vi "Curtin1_Plot.vi"(5 "Canvas 2":refnum<vi>, 6 "Force YRescale":bool, 7 "Settings":T2 {"mag/phase" items=["FRF", "rad phase unwrapped", "deg phase unwrapped", "rad phase wrapped", "deg phase wrapped", "White Plots", "MJ Map", "Real and Imaginary"]; "Bands" items=["No Bands", "", "Test2", "test3", "Test"]; "Smoothing" items=["No smoothing"=0, "1/4 semitone"=25, "1/2 semitone"=50, "1 semitone"=100, "2 semitones"=200, "Woodhouse"=19]; "View Type" items=["As measured", "Normalize", "Separate", "Complex Average", "Real Average", "Standard Deviation"]}, 8 "VI Refnum":refnum<vi>, 10 "Files":T3[](array[typedef]), 11 "FRF":refnum<vi>) -> (0 "Complex Out":cluster{dbl, "df":dbl, cdb[]}[](array[cluster]), 1 "size(s)":i32, 2 "Average FRF":cluster{"x0":dbl, "df":dbl, dbl[]}[](graph), 3 "MJ Plot":dbl[][](graph))   [LabVIEW 2022 SP3]
uses:
  Mic/Mic_Global.vi
  Curtin1_Label.ctl
  GraphType.ctl
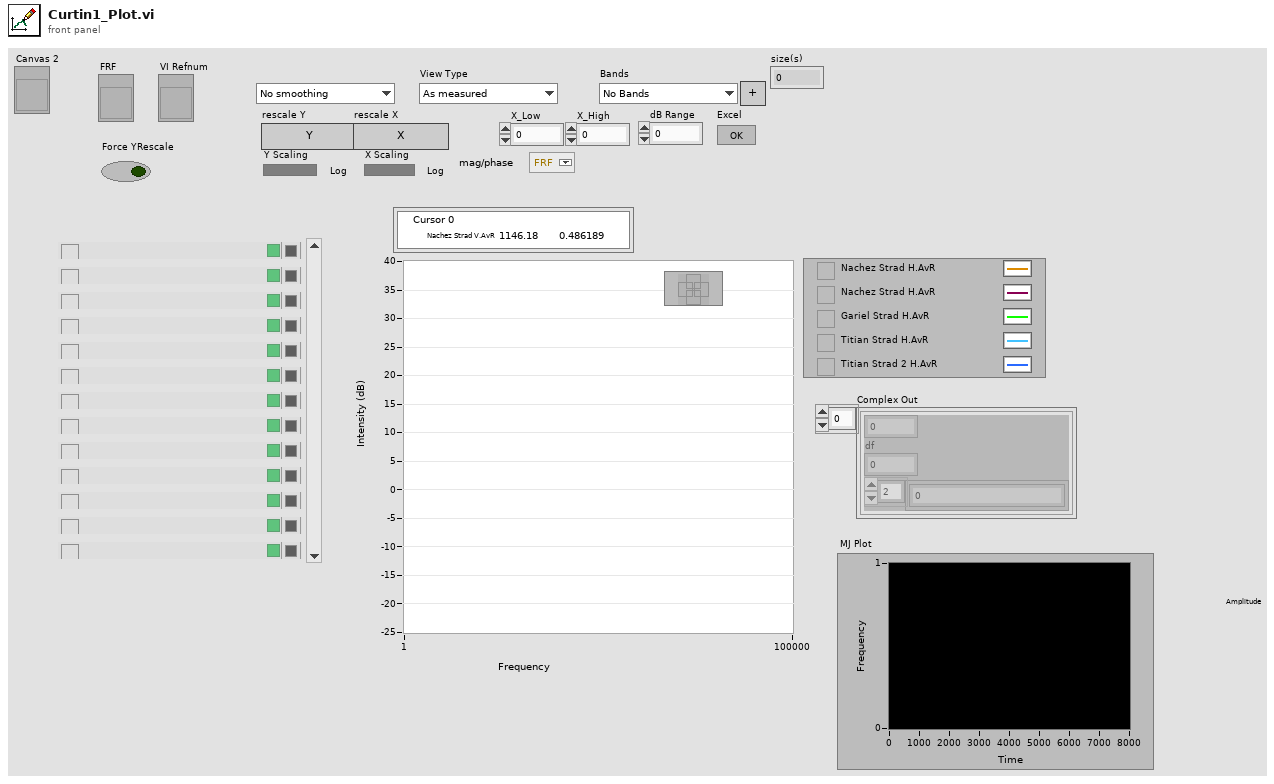
[diagram p1: front panel]
types:
  T1 = typedef "GraphType.ctl" = u16
  T2 = cluster{"View Type":u16, "Smoothing":u16, "Bands":u16, "New Band":bool, "rescale Y":bool, "rescale X":bool, "X_Low":dbl, "X_High":dbl, "dB Range":dbl, "Excel":bool, "Y Scaling":bool, "X Scaling":bool, "mag/phase":T1}
  T3 = typedef "Curtin1_Label.ctl" = cluster{"Show?":bool, "Name":string, "Color":u32, "Path":path, "Show Notes":bool, "correlate":bool}
  T4 = typedef "LVBoundsTypeDef.ctl" = cluster{"Width":u32, "Height":u32}
  T5 = typedef "PreferencesControl.ctl" = cluster{"Name of test":string, "Date":timestamp, "Location":string, "Template":string, "Soundcard":string, "resolution":u16, "Sampling rate":u16, "Ch1 Gain ":dbl, "Ch2 Gain":dbl, "Sample time (s)":dbl, "Pre-trigger (s)":dbl, "Hammer Threshold":dbl, "Positions":i16, "Taps/Position":i16, "Set Names":string, "Freq resolution":dbl, "Hammer cutoff":dbl, "Mic cutoff":dbl, "Double bounce ":dbl, "Hammer Cal":dbl, "dB Offset":dbl, "Accel Cal":dbl, "Vibrometer Cal":dbl, "Mic Cal":dbl, "Output":u16, "Voltage Cal":dbl, "Vibrometer Port":refnum<visa-resource-name>, "Range":u16, "High Pass":u16, "Bandwidth":u16, "X Range":cluster{"Minimum":dbl, "Maximum":dbl, "Increment":dbl, "Minor Increment":dbl, "Start":dbl}[], "Y Range":cluster{"Minimum":dbl, "Maximum":dbl, "Increment":dbl, "Minor Increment":dbl, "Start":dbl}[], "dB Spread":dbl, "Trigger":u16, "Ch_1":u8, "Ch_2":u8, "flip?":bool, "60Hz":bool, "Time offset":dbl, "Piezo Cal":dbl, "Default Notes":string, "Tom":bool}
  T6 = cluster{"Alerts":bool, "Log X Axis":bool, "dB scale":bool, "Averaging":bool, "Fade":dbl, "Centroids?":bool, "line thickness":u8}
  T7 = cluster{dbl, "df":dbl, "Power Spectrum (V^2 rms)":dbl[]}[]
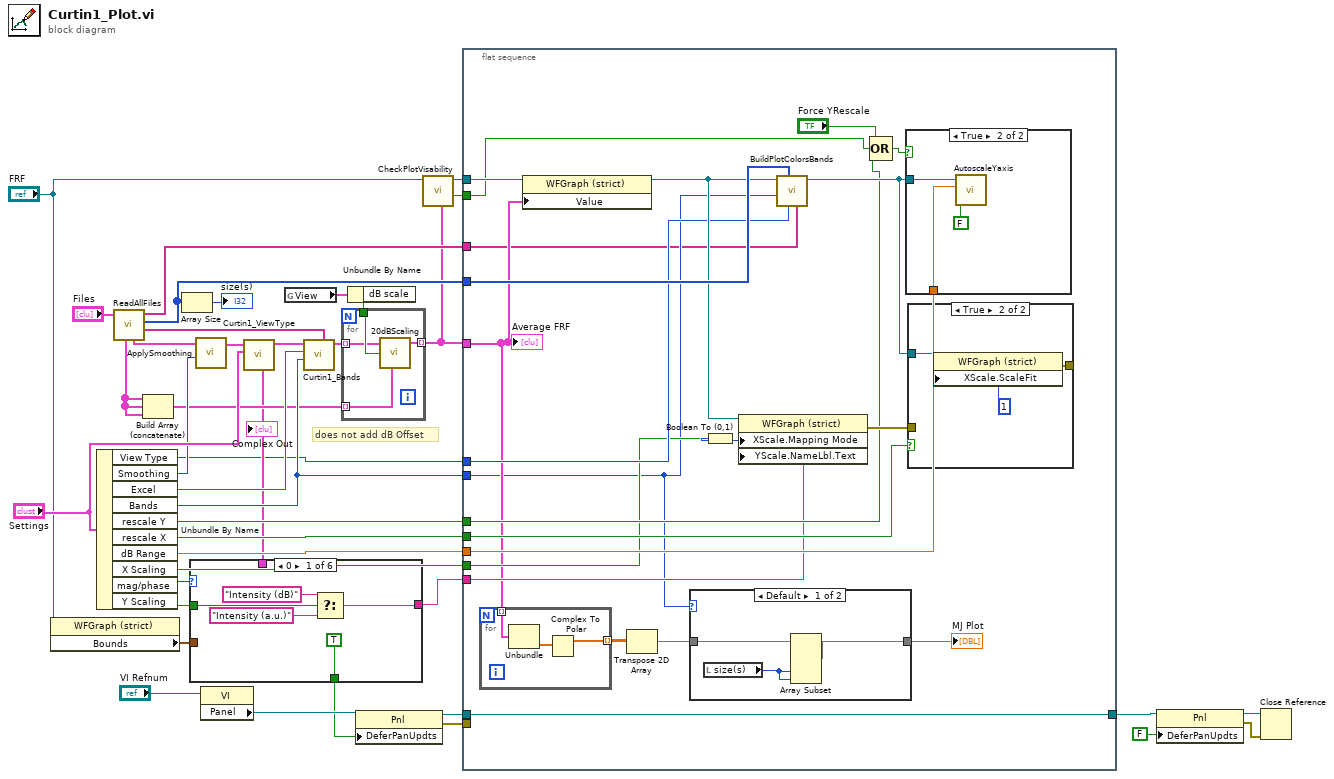
[diagram p0: block diagram]
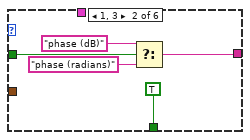
[diagram p2: hidden frame]
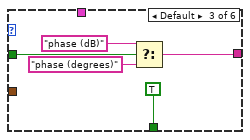
[diagram p3: hidden frame]
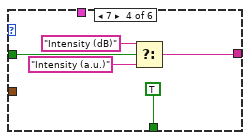
[diagram p4: hidden frame]
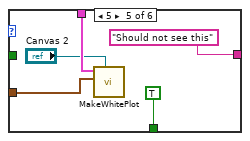
[diagram p5: hidden frame]
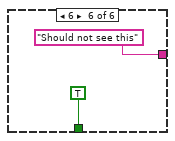
[diagram p6: hidden frame]
diagram:
  # "does not add dB Offset"
  n1 = property class="WFGraph (strict)"(reference="FRF") -> ("Bounds"=w4:T4)  [unwired: 1 in, 2 out]
  n2 = Unbundle By Name("Settings") -> ("View Type"=w2:u16, "Smoothing"=w22:u16, "Excel"=w20:bool, "Bands"=w21:u16, "rescale Y"=w26:bool, "rescale X"=w25:bool, "dB Range"=w23:dbl, "X Scaling"=w12:bool, "mag/phase"=w11:T1, "Y Scaling"=w10:bool)
  n3 = call "ReadAllFiles.vi"("Files"="Files") -> ("Selected Names"=w18:string[], "selected colors"=w17:u32[], "All Names"=w19:string[], "data"=w33:cluster{"t0":dbl, "df":dbl, "Y":cdb[]}[], "Settings"=w8:T5[])  [unwired: 5 in, 1 out]
  n4 = Build Array (concatenate)(w8, w8, w8) -> (w7:T5[])
  n5 = Array Size(array=w17) -> (size(s)=→"size(s)":i32)
  n6 = call "ApplySmoothing.vi"("Smoothing"=w22, "Complex FRF"=w33) -> ("Complex FRF Out"=w32:cluster{dbl, "df":dbl, cdb[]}[])  [unwired: 9 in]
  n7 = property class="VI"(reference="VI Refnum") -> ("Panel"=w40:refnum<vi>)  [unwired: 1 in, 2 out]
  n8 = call "Curtin1_ViewType.vi"("Settings"="Settings", "FRF in"=w32) -> ("Complex Out"=w6:cluster{dbl, "df":dbl, cdb[]}[], "FRF Out"=w31:cluster{"x0":dbl, "df":dbl, dbl[]}[])  [unwired: 8 in]
  "Complex Out" <- w6
  n9 = case shown="0" w11 {
    tunnel: w10 -> [w43 w48 w53 w58 _ _]
    tunnel: [w42 w47 w52 w57 "Should not see this" ("Position") "Should not see this" ("Position")] -> w9
    tunnel: w6 -> [_ _ _ _ w64 _]
    tunnel: w4 -> [_ _ _ _ w63 _]
    tunnel: [TRUE ("Defer Panel Updates") TRUE ("Defer Panel Updates") TRUE ("Defer Panel Updates") TRUE ("Defer Panel Updates") TRUE ("Defer Panel Updates") TRUE ("Defer Panel Updates")] -> w3
    frame 0 {
      n10 = Select(t="Intensity (dB)" ("Position"), s=w43, f="Intensity (a.u.)" ("Position")) -> (s? t:f=w42:string)
    }
    frame 1, 3 {
      n11 = Select(t="phase (dB)" ("Position"), s=w48, f="phase (radians)" ("Position")) -> (s? t:f=w47:string)
    }
    frame Default {
      n12 = Select(t="phase (dB)" ("Position"), s=w53, f="phase (degrees)" ("Position")) -> (s? t:f=w52:string)
    }
    frame 7 {
      n13 = Select(t="Intensity (dB)" ("Position"), s=w58, f="Intensity (a.u.)" ("Position")) -> (s? t:f=w57:string)
    }
    frame 5 {
      n14 = call "MakeWhitePlot.vi"("Canvas"="Canvas 2", "Bounds"=w63, "Complex In"=w64) -> ()  [unwired: 8 in, 1 out]
    }
    frame 6 {
    }
  }
  n15 = global read "Mic_Global.vi" "View"() -> (w29:T6)
  n16 = call "Curtin1_Bands.vi"("File Names"=w18, "Bands"=w21, "Excel?"=w20, "Magnitude"=w31) -> ("Filter"=w27:T7)  [unwired: 6 in, 1 out]
  n17 = Unbundle By Name(w29) -> ("dB scale"=w28:bool)
  n18 = for {
    tunnel: w28 -> [w71]
    tunnel: w27 -> [w70] mode=indexing
    tunnel: [w69] -> w14 mode=indexing
    tunnel: w7 -> [w68] mode=indexing
    n19 = call "20dBScaling.vi"("Average FRF in"=w70, "dB?"=w71, "Settings"=w68) -> ("Average FRF out"=w69:cluster{"x0":dbl, "df":dbl, dbl[]})  [unwired: 3 in, 1 out]
  }
  n20 = property class="Pnl"(reference=w40, "DeferPanUpdts"=w3) -> (reference out=w36:refnum<vi>, error out=w30:errorcluster)  [unwired: 1 in]
  n21 = call "CheckPlotVisability.vi"("Array"=w14, "WaveformGraph in"="FRF") -> ("rescale"=w13:bool, "WaveformGraph out"=w15:refnum<vi>)  [unwired: 8 in]
  n22 = flat-sequence {
    tunnel: w17 -> [w87]
    tunnel: w15 -> [w91]
    tunnel: w14 -> [w77]
    tunnel: [w93] -> w37
    tunnel: w36 -> [w93]
    tunnel: w30 -> [_]
    tunnel: w19 -> [w72]
    tunnel: w26 -> [w82]
    tunnel: w25 -> [w90]
    tunnel: w23 -> [w88]
    tunnel: w21 -> [w75]
    tunnel: w2 -> [w85]
    tunnel: w13 -> [w83]
    tunnel: w12 -> [w80]
    tunnel: w9 -> [w78]
    frame #0 {
      n23 = for {
        tunnel: w77 -> [w99] mode=indexing
        tunnel: [w98] -> w76 mode=indexing
        n24 = Unbundle(w99) -> (w100:dbl[])  [unwired: 2 out]
        n25 = Complex To Polar(r * e^(i*theta)=w100) -> (r=w98:dbl[])  [unwired: 1 out]
      }
      n26 = property class="WFGraph (strict)"(reference=w91, "Value"=w77) -> (reference out=w86:refnum<vi>)  [unwired: 1 in, 1 out]
      n27 = Transpose 2D Array(2D array=w76) -> (transposed array=w73:dbl[][])
      n28 = case shown="Default" w75 {
        tunnel: [w94 w97] -> w74
        tunnel: w73 -> [w96 w97]
        frame Default {
          n29 = local read "size(s)"() -> (w95:i32)
          n30 = Array Subset(array=w96, index (col)=w95, length (col)=w95) -> (w94:dbl[][])  [unwired: 2 in]
        }
        frame 0 {
        }
      }
      "MJ Plot" <- w74
      n31 = Boolean To (0,1)(Boolean=w80) -> (0, 1=w92:i16)
      n32 = property on="Property Node" class="WFGraph (strict)"(reference=w86, "XScale.Mapping Mode"=w92, "YScale.NameLbl.Text"=w78) -> (error out=w84:errorcluster)  [unwired: 1 in, 1 out]
      n33 = call "BuildPlotColorsBands.vi"("Labels"=w72, "View Type"=w85, "Colors"=w87, "Bands"=w75, "WaveformGraph in"=w86) -> ("WaveformGraph out"=w89:refnum<vi>)  [unwired: 6 in]
      n34 = Compound Arithmetic op=OR("Force YRescale", w83, w82) -> (w81:bool)
      n35 = case shown="True" w81 {
        tunnel: w89 -> [_ w106]
        tunnel: w88 -> [_ w105]
        frame False {
        }
        frame True {
          n36 = call "AutoscaleYaxis.vi"("Has Coherence in plot?"=FALSE, "dB Range"=w105, "WaveformGraph in"=w106) -> ()  [unwired: 9 in]
        }
      }
      n37 = case shown="True" w90 {
        tunnel: w89 -> [_ w103]
        tunnel: [_ w101] -> _
        tunnel: w84 -> [_ _]
        frame False {
        }
        frame True {
          n38 = property class="WFGraph (strict)"(reference=w103, "XScale.ScaleFit"=u8 1 ("Y Scale.Scale Fit")) -> (error out=w101:errorcluster)  [unwired: 1 in, 1 out]
        }
      }
      "Average FRF" <- w77
    }
  }
  n39 = property class="Pnl"(reference=w37, "DeferPanUpdts"=FALSE ("Defer Panel Updates")) -> (reference out=w34:refnum<vi>, error out=w35:errorcluster)  [unwired: 1 in]
  n40 = Close Reference(reference=w34, error in (no error)=w35) -> ()  [unwired: 1 out]
